vi "E727_Setup IV.vi"(0 "On/Off":bool, 1 "Move to middle?":bool, 2 "Perform autozero?":bool, 3 "error in":errorcluster) -> (7 "Conn. Axis":string[](array[string]), 8 "Running":bool caption="Configuration_Setup.vi is running", 10 "error out":errorcluster)   [LabVIEW 2022 SP3]
panel:
  out "Interface":u16(ring) items=["RS232", "TCP/IP", "USB"]
  out "USB settings":cluster{"S/N":string, "USB Search?":bool}={"S/N"="", "USB Search?"=TRUE}
  out "Identification":string
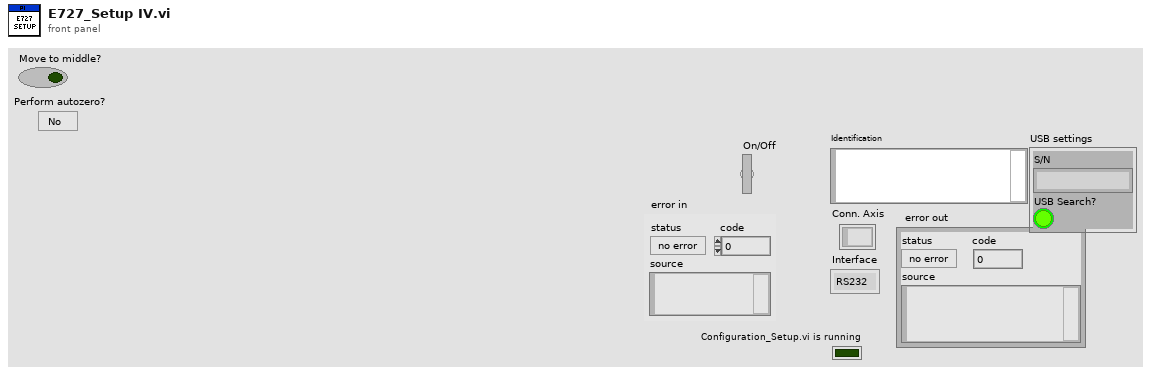
[diagram p1: front panel]
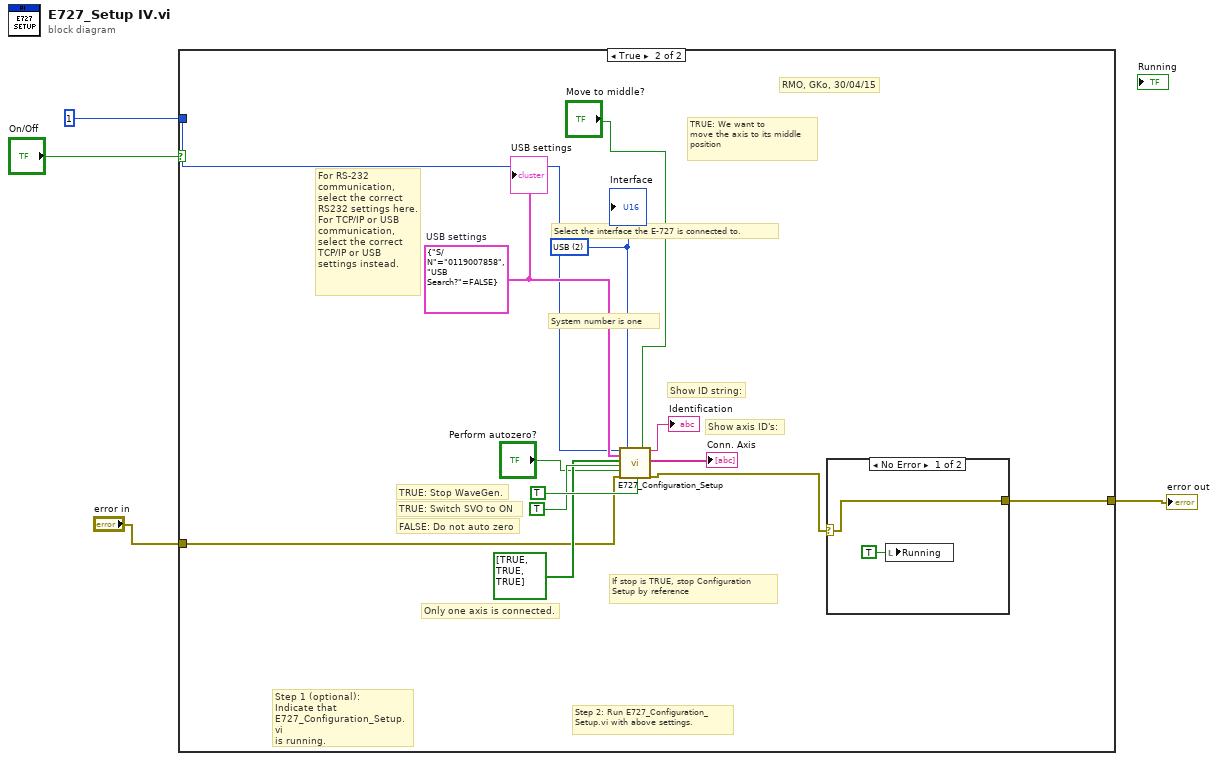
[diagram p0: block diagram]
diagram:
  n1 = case shown="True" "On/Off" {
    tunnel: 1 ("System no.") -> [_ w13]
    tunnel: "error in" -> [w5 w11]
    tunnel: [w5 w8] -> w2
    frame False {
    }
    frame True {
      w14 = cluster{"S/N":string, "USB Search?":bool} {"S/N"="0119007858", "USB Search?"=FALSE}  # USB settings
      w12 = u16 2 items=["RS232", "TCP/IP", "USB"] ("Interface")
      # "Only one axis is connected."
      # "TRUE: We want to\nmove the axis to its middle\nposition"
      # "FALSE: Do not auto zero"
      # "TRUE: Switch SVO to ON"
      # "If stop is TRUE, stop Configuration\nSetup by reference"
      # "For RS-232 \ncommunication,\nselect the correct\nRS232 settings here.\nFor TCP/IP or USB \ncommunication, \nselect the correct \nTCP/IP or USB\nsettings instead."
      # "Select the interface the E-727 is connected to."
      # "RMO, GKo, 30/04/15"
      # "Step 2: Run E727_Configuration_\nSetup.vi with above settings."
      # "Step 1 (optional): \nIndicate that\nE727_Configuration_Setup.vi\nis running."
      # "Show axis ID's:"
      # "Show ID string:"
      # "TRUE: Stop WaveGen."
      # "System number is one"
      n2 = call "E727_Configuration_Setup.vi"("System no."=w13, "USB settings"=w14, "Are stages connected?"=bool[] [TRUE, TRUE, TRUE], "Change servo status to ON?"=TRUE ("Use dialog to define\nconnected stages?"), "Perform autozero?"="Perform autozero?", "error in"=w11, "Interface"=w12, "Stop wave generator\noutput (if any)"=TRUE ("All axes?"), "Move to middle?"="Move to middle?") -> ("Identification"=→"Identification":string, "All conn. axes"=→"Conn. Axis":string[], "error out"=w9:errorcluster)  [unwired: 5 in, 3 out]
      n3 = case shown="No Error" w9 {
        selector: w9 -> [w20 w21]
        tunnel: [w20 w21] -> w8
        frame No Error {
          n4 = local write "Running"(TRUE ("Running")) -> ()
        }
        frame Error {
        }
      }
      "USB settings" <- w14
      "Interface" <- w12
    }
  }
  "error out" <- w2
